vi "Voltage - Continuous HW Timed Output-Adj.vi"() -> ()   [LabVIEW 2014]
doc: "This example demonstrates how to continuously re-generate analog output data from a buffer in your computer's memory.\n\nRefer to your device documentation for pinouts and hardware capabilities."
uses:
  <vilib>/Utility/error.llb/DialogType.ctl
  <vilib>/DAQmx/create/channels.llb/DAQmx Create Channel (AO-Voltage-Basic).vi
  <vilib>/DAQmx/configure/timing.llb/DAQmx Timing (Sample Clock).vi
  <vilib>/DAQmx/write.llb/DAQmx Write (Analog 1D Wfm NChan NSamp).vi
  <resource>/objmgr/daqmx.rc
  <vilib>/measure/NI_MABase.lvlib
panel:
  in  "Output Array":T1(array[cluster])=[{"Waveform Type"=0, "Amplitude"=1.0, "Frequency"=10.0}] {"Frequency" format="%0.2p"; "Amplitude" format="%0.2p"; "Waveform Type" items=["Sine Wave", "Triangle Wave", "Square Wave", "Sawtooth Wave"]}
  in  "Number of Samples":i32=1000
  in  "Stop":bool
  out "Waveform Graph":waveform(dbl)[](graph)=[{"t0"=timestamp(0 s since 1904-01-01), "dt"=0.001, "Y"=[]}]
  in  "Sample Rate":dbl=1000.0
  in  "Sample Clock Source":tag="OnboardClock"
  in  "Max Voltage":dbl=5.0
  in  "Min Voltage":dbl=-5.0
  in  "Physical Channel(s)":tag="Dev1/ao0"
  out "Actual Sample Rate":dbl=1000.0 format="%0.2f"
  # "Channel Settings"
  # "Output"
  # "Timing and Buffer Settings"
  # "Waveform Settings"
  # "The number of elements in the waveform array must equal the number of channels in the task."
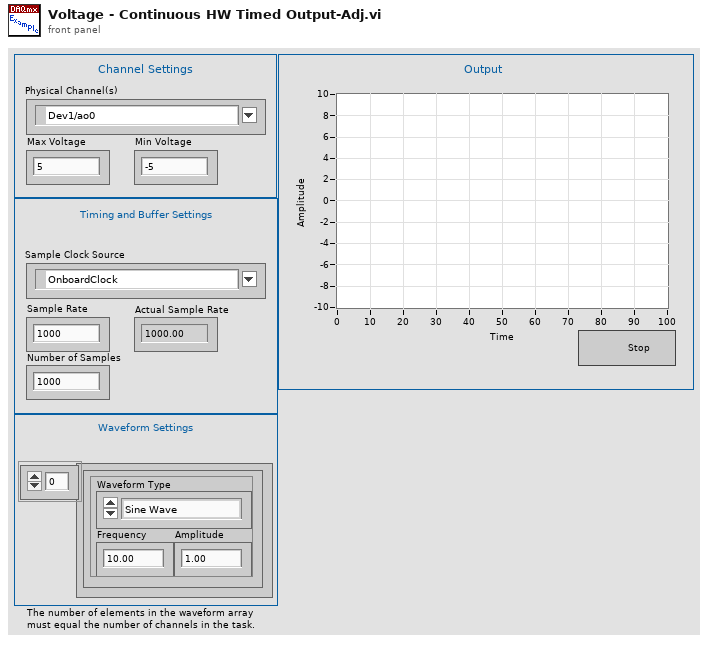
[diagram p1: front panel]
types:
  T1 = cluster{"Waveform Type":u16, "Amplitude":dbl, "Frequency":dbl}[]
  T2 = typedef "DialogType.ctl" = u16
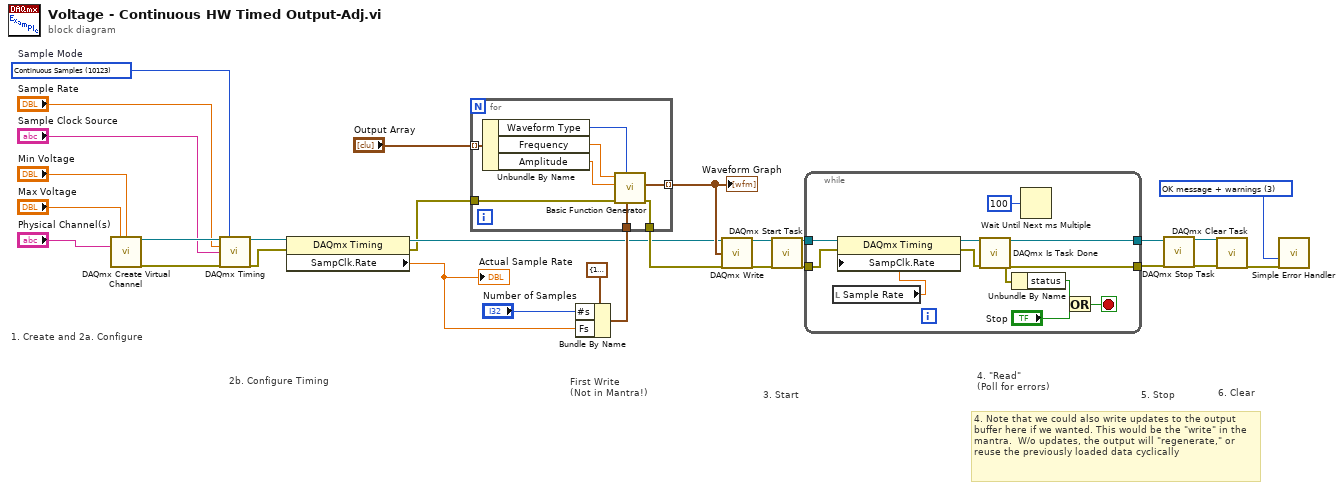
[diagram p0: block diagram]
diagram:
  w6 = T2 3 items=["no dialog", "OK message", "continue or stop message", "OK message + warnings", "continue/stop + warnings"] ("type of dialog (OK msg:1)")
  w27 = 10123 items=["Finite Samples"=10178, "Continuous Samples"=10123, "Hardware Timed Single Point"=12522]  # Sample Mode
  # "6. Clear"
  # "5. Stop"
  # "4. Note that we could also write updates to the output buffer here if we wanted. This would be the \"write\" in the mantra.  W/o updates, the output will \"regenerate,\" or reuse the previously loaded data cyclically"
  # "4. \"Read\"\n(Poll for errors)"
  # "3. Start"
  # "First Write\n(Not in Mantra!)"
  # "2b. Configure Timing"
  # "1. Create and 2a. Configure"
  n1 = call-poly <vilib>:"DAQmx Create Virtual Channel.vi"("maximum value"="Max Voltage", "minimum value"="Min Voltage", "physical channels"="Physical Channel(s)") -> ("task out"=w25:refnum<k21>, "error out"=w26:errorcluster)  [unwired: 11 in]
  n2 = call-poly <vilib>:"DAQmx Timing.vi"("task/channels in"=w25, "sample mode"=w27, "rate"="Sample Rate", "source"="Sample Clock Source", "error in"=w26) -> ("task out"=w29:refnum<k21>, "error out"=w28:errorcluster)  [unwired: 9 in]
  n3 = property class="DAQmx Timing"(reference=w29, error in=w28) -> (reference out=w5:refnum<k21>, error out=w4:errorcluster, "SampClk.Rate"=w1:dbl)
  "Actual Sample Rate" <- w1
  n4 = Bundle By Name(cluster=cluster{"Fs":dbl, "#s":dbl} {"Fs"=1000.0, "#s"=1000.0} ("sampling info"), "#s"="Number of Samples", "Fs"=w1) -> (w16:cluster{"Fs":dbl, "#s":dbl})
  n5 = for {
    tunnel: w4 -> [w37]
    tunnel: w16 -> [w36]
    tunnel: [w35] -> w13
    tunnel: "Output Array" -> [w34] mode=indexing
    tunnel: [w30] -> w11 mode=indexing
    n6 = Unbundle By Name(w34) -> ("Waveform Type"=w33:u16, "Frequency"=w32:dbl, "Amplitude"=w31:dbl)
    n7 = call <vilib>:"Basic Function Generator.vi"("sampling info"=w36, "signal type"=w33, "error in (no error)"=w37, "amplitude"=w31, "frequency"=w32) -> ("error out"=w35:errorcluster, "signal out"=w30:waveform(dbl))  [unwired: 4 in, 1 out]
  }
  "Waveform Graph" <- w11
  n8 = call-poly <vilib>:"DAQmx Write.vi"("task/channels in"=w5, "data"=w11, "error in"=w13) -> ("task out"=w15:refnum<k21>, "error out"=w14:errorcluster)  [unwired: 10 in, 1 out]
  n9 = call <vilib>:"DAQmx Start Task.vi"("task/channels in"=w15, "error in"=w14) -> ("task out"=w24:refnum<k21>, "error out"=w23:errorcluster)  [unwired: 12 in]
  n10 = while {
    tunnel: w24 -> [w48]
    tunnel: w23 -> [w40]
    tunnel: [w45] -> w7
    tunnel: [w46] -> w8
    stop <- w47 stop-if-true
    n11 = local read "Sample Rate"() -> (w38:dbl)
    n12 = property class="DAQmx Timing"(reference=w48, error in=w40, "SampClk.Rate"=w38) -> (reference out=w41:refnum<k21>, error out=w39:errorcluster)
    n13 = call <vilib>:"DAQmx Is Task Done.vi"("task/channels in"=w41, "error in"=w39) -> ("task out"=w46:refnum<k21>, "error out"=w45:errorcluster)  [unwired: 11 in, 1 out]
    n14 = Unbundle By Name(w45) -> ("status"=w44:bool)
    n15 = Wait Until Next ms Multiple(millisecond multiple=u32 100) -> ()  [unwired: 1 out]
    n16 = Or(x=w44, y="Stop") -> (x .or. y?=w47:bool)
  }
  n17 = call <vilib>:"DAQmx Stop Task.vi"("task/channels in"=w8, "error in"=w7) -> ("task out"=w10:refnum<k21>, "error out"=w9:errorcluster)  [unwired: 12 in]
  n18 = call <vilib>:"DAQmx Clear Task.vi"("task in"=w10, "error in"=w9) -> ("error out"=w22:errorcluster)  [unwired: 13 in]
  n19 = call <vilib>:"Simple Error Handler.vi"("type of dialog (OK msg:1)"=w6, "error in (no error)"=w22) -> ()  [unwired: 3 in, 5 out]
